vi "LoadFromINI.vi"(8 "error in (no error)":errorcluster, 10 "path":path, 11 "reference in":refnum<class "niMmWave_Reciever.lvclass">) -> (0 "error out":errorcluster, 3 "reference out":refnum<class "niMmWave_Reciever.lvclass">)   [LabVIEW 2019, in "niMmWave_Reciever.lvclass"]
doc: "Loads insturment data from ini file"
uses:
  niMmWave_Reciever.lvclass
  <vilib>/Utility/error.llb/Error Cluster From Error Code.vi
  <vilib>/Utility/config.llb/Read Key (String).vi
  <vilib>/ErrorRing/Error Ring.xnode
  <vilib>/Utility/config.llb/NI_LVConfig.lvlib
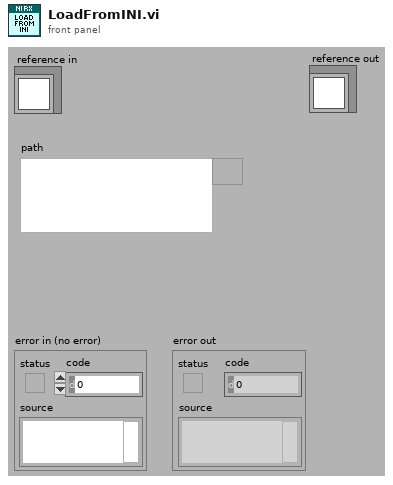
[diagram p1: front panel]
types:
  T1 = cluster{"IF":string, "RX_ADC":string, "RX_FPGA":string}
  T2 = typedef "niMmWave_Reciever.lvclass/ObjectAttributesRef.ctl" = refnum<data-value>
  T3 = typedef "NI_LVConfig.lvlib/Config Data RefNum.ctl" = refnum<k1>
  T4 = typedef "niMmWave_Reciever.lvclass/ObjectAttributes.ctl" = cluster{"session":T5[], "HW.RX devices":T19, "RF config":T20, "RX trigger options":T21, "RX samples":i32, "RX Fs":dbl}
  T5 = typedef "Session.ctl" = cluster{"3620 session":refnum<queue>, "tx baseband session":T6, "rx baseband session":T14, "tx gain (dB)":dbl, "rx gain (dB)":dbl, "hardware configuration":T15, "gain ranging":T17[], "pxi trigger bus information":T18}
  T6 = typedef "Tx Baseband Session.ctl" = cluster{"3610 session":T7, "7902 reference":T13}
  T7 = typedef "ni3610_and_ni3630_Driver_Lib.lvlib/Main Settings.ctl" = cluster{"VISA resource name":refnum<visa-resource-name>, "Address Space":T8, "window_offset":u32, "register_addresses":T9, "required_MM_fpga_version":cluster{"signature":u32, "hardware":u32, "current revision":u32, "oldest revision":u32}, "CPLD Oldest Compat Version ":cluster{"hardware":u32, "CPLD firmware":u32}, "MM_FPGA_image_location":string, "is_init":bool, "card_type":T10, "DacLmkConfigFileName":string, "AdcLmkConfigFileName":string, "AdcConfigFileName":string, "DacConfigFileName_RevA":string, "DacConfigFileName_RevB":string, "Mulde hardware revision":u8, "bypass DAC PLL\n":bool, "IQ Card Revision":T11, "board capability":T12}
  T8 = typedef "VISA Register Access Address Space.ctl" = u16
  T9 = typedef "ni3610_and_ni3630_Driver_Lib.lvlib/Register Adresses.ctl" = cluster{"MM based Registers":cluster{"Revision":u32, "OldestCompatRev":u32, "signature":u32, "scratch":u32, "LedControl":u32, "BoardHwRev":u32, "BoardControl":u32, "ThermalStatus":u32, "BasebandStatus":u32, "BasebandControl":u32, "BasebandAuxSetup":u32, "BasebandAuxStatus":u32, "LmkSyncOutSetup":u32, " AdcSyncOutSetup":u32, " InjSyncOutSetup":u32, " PxiTrig0OutSetup":u32, " PxiTrig1OutSetup":u32, " PxiTrig2OutSetup":u32, " PxiTrig3OutSetup":u32, " PxiTrig4OutSetup":u32, " PxiTrig5OutSetup":u32, " PxiTrig6OutSetup":u32, " PxiTrig7OutSetup":u32}, "CPLD based Registers":cluster{"SlaveSignature":u32, "SlaveRevision":u32, "SlaveOldestCompatRev":u32, "SlaveScratch":u32, "SlaveSetup":u32, "SlaveStatus":u32, "IDacReg_offset":u32, "LMKRegGrp0_offset":u32, "QDacReg_offset":u32, "BrdTempSensorVal":u32, "TempSensorPowerDown":u32, "GPIOReg_offset":u32, "IAdcReg_offset":u32, "QAdcReg_offset":u32, "LMKRegGrp1_offset":u32, "QadcTempSensorVal":u32, "IadcTempSensorVal":u32, "RevisionReg":u32, "VcxoReg":u32, "CpldStatusReg":u32, "PowerReg":u32, "VBiasEnReg":u32, "ExtRefOeReg":u32, "QdacCtrlReg":u32, "QdacStatusReg":u32, "IdacCtrlReg":u32, "IdacStatusReg":u32, "QdacJtagIn":u32, "QdacJtagOut":u32, "IdacJtagIn":u32, "IdacJtagOut":u32, "IqDcSetupReg":u32, "QadcStatusReg":u32, "IadcStatusReg":u32, "BrdSetupReg":u32, "IqDcRevisionReg":u32, "PllStatusReg":u32, "EndpointScratchReg":u32, "AdcSyncCfgReg":u32, "IqCardOpampReg":u32}, "CPLD Register Offset":u32, "MM  Register Offset":u32, " PxiTrig0OutSetup":u32}
  T10 = typedef "ni3610_and_ni3630_Driver_Lib.lvlib/Base Card Type.ctl" = enum16{"unspecified", "ADC", "DAC"}
  T11 = typedef "ni3610_and_ni3630_Driver_Lib.lvlib/IQ Card Revision.ctl" = enum16{"RevA", "RevB", "RevC", "RevD"}
  T12 = typedef "ni3610_and_ni3630_Driver_Lib.lvlib/Board Capability.ctl" = cluster{"baseband sync":enum16{"no baseband sync", "baseband sync"}}
  T13 = typedef "Blank FPGA Reference.ctl" = refnum<k20>
  T14 = typedef "Rx Baseband Session.ctl" = cluster{"3630 session":T7, "7902 reference":T13}
  T15 = typedef "Hardware Configuration.ctl" = cluster{"direction":T16, "baseband only":bool}
  T16 = typedef "Direction.ctl" = enum16{"Transceiver", "Receiver", "Transmitter"}
  T17 = typedef "Gain Ranging.ctl" = cluster{"gain ranging active scope":string, "gain ranging stream session":refnum<k20>}
  T18 = typedef "PXI Trigger Bus Info.ctl" = cluster{"chassis resource name":refnum<visa-resource-name>, "7902R (TX)":i16, "3610 (TX)":i16, "3620 (IF)":i16, "3630 (RX)":i16, "7902R (RX)":i16}
  T19 = typedef "mmWave HW Control.lvlib/HW RX resources cluster.ctl" = cluster{"HW.IF":tag, "HW.ADC":refnum<visa-resource-name>, "HW.RX FPGA":tag}
  T20 = typedef "mmWave HW Control.lvlib/HW RX RF config cluster.ctl" = cluster{"Gain":dbl, "Frequency":dbl, "mmWave adapter":string}
  T21 = typedef "TX trigger config.ctl" = cluster{"delay":dbl, "trig source":T22, "PXI src":i32, "export":T23, "PXI dest":i32}
  T22 = typedef "FPGA Utility.lvlib/FPGA driver trigger source.ctl" = enum16{"Use Tclk", "PXI_Trig", "Aurora RX trig"}
  T23 = typedef "FPGA Utility.lvlib/FPGA driver trigger destination.ctl" = enum16{"None", "Source trig", "Synced trig", "Delayed sync"}
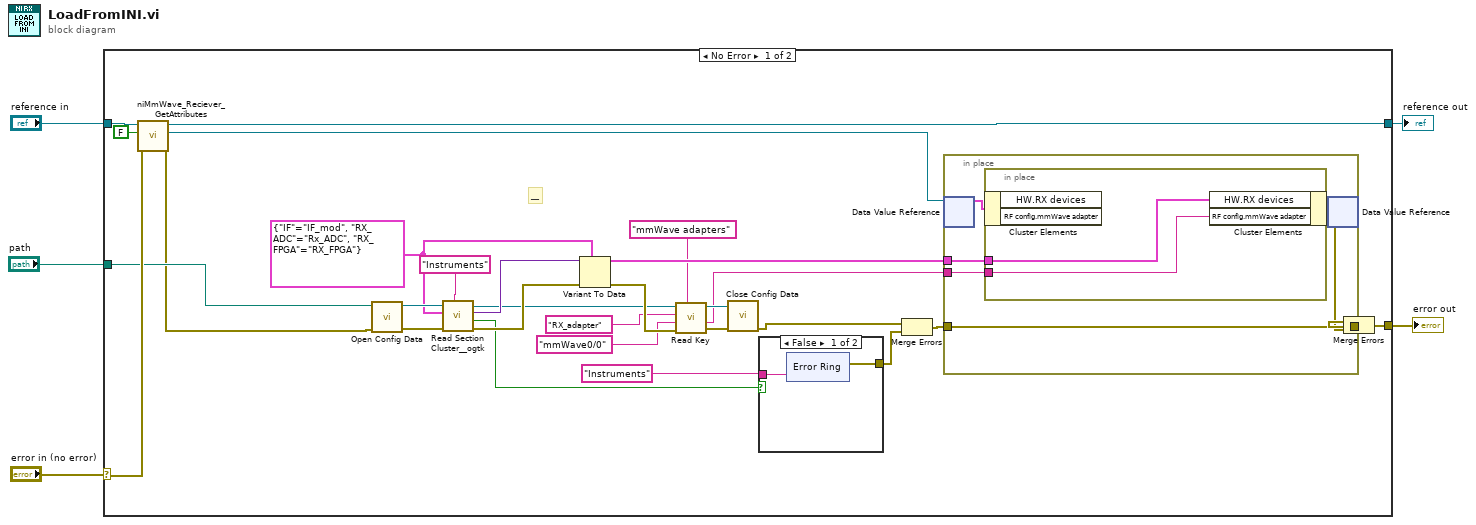
[diagram p0: block diagram]
diagram:
  n1 = case shown="No Error" "error in (no error)" {
    selector: "error in (no error)" -> [w32 w53]
    tunnel: [w35 w53] -> w4
    tunnel: [w33 w52] -> w2
    tunnel: "reference in" -> [w34 w52]
    tunnel: "path" -> [w21 _]
    frame No Error {
      w22 = T1 {"IF"="IF_mod", "RX_ADC"="Rx_ADC", "RX_FPGA"="RX_FPGA"} ("HW.RX resources")
      # "__"
      n2 = call "niMmWave_Reciever_GetAttributes.vi"("error in (no error)"=w32, "return data? (T)"=FALSE, "reference in"=w34) -> ("error out"=w14:errorcluster, "attributes ref"=w29:T2, "reference out"=w33:refnum<class "niMmWave_Reciever.lvclass">)  [unwired: 5 in, 1 out]
      n3 = call <vilib>:"Open Config Data.vi"("error in (no error)"=w14, "configuration file path"=w21) -> ("error out"=w26:errorcluster, "refnum"=w27:T3)  [unwired: 7 in, 1 out]
      n4 = call <userlib>:"Read Section Cluster__ogtk.vi"("section (optional)"="Instruments", "error in (no error)"=w26, "Section Formatted Cluster Type"=w22, "refnum"=w27) -> ("error out"=w24:errorcluster, "all found?"=w20:bool, "Section Formatted Cluster"=w25:variant, "dup refnum"=w11:T3)  [unwired: 3 in, 1 out]
      n5 = Variant To Data(error in=w24, type=w22, Variant=w25) -> (data=w17:T1, error out=w13:errorcluster)
      n6 = call-poly <vilib>:"Read Key.vi"("section"="mmWave adapters" ("section (optional)"), "error in (no error)"=w13, "default value"="mmWave0/0" ("section (optional)"), "key"="RX_adapter" ("section (optional)"), "refnum"=w11) -> ("error out"=w8:errorcluster, "value"=w7:string, "refnum out"=w9:T3)  [unwired: 3 in, 1 out]
      n7 = call <vilib>:"Close Config Data.vi"("error in (no error)"=w8, "refnum"=w9) -> ("error out"=w16:errorcluster)  [unwired: 8 in, 1 out]
      n8 = case shown="False" w20 {
        tunnel: "Instruments" ("section (optional)") -> [w44 _]
        tunnel: [w43 _] -> w18
        frame False {
          n9 = xnode "Error Ring"("parameter 0"=w44) -> ("error out"=w43:errorcluster)
        }
        frame True {
        }
      }
      n10 = Merge Errors(w16, w18) -> (w15:errorcluster)
      n11 = in-place {
        in-place-border: w15 -> [w38]
        in-place-border: [w38] -> w31
        in-place-border: w17 -> [w37]
        in-place-border: w7 -> [w36]
        n12 = in-place-dvr #1(w29) -> (w39:T4)  [unwired: 1 out]
        n13 = in-place {
          in-place-border: w37 -> [w42]
          in-place-border: w36 -> [w41]
          n14 = in-place-cluster #2(w39) -> ()  [unwired: 2 out]
          n15 = in-place-cluster #2("HW.RX devices"=w42, "RF config.mmWave adapter"=w41) -> (w40:T4)
        }
        n16 = in-place-dvr #1(w40) -> (w30:errorcluster)  [unwired: 1 out]
      }
      n17 = Merge Errors(w31, w30) -> (w35:errorcluster)
    }
    frame Error {
    }
  }
  "error out" <- w4
  "reference out" <- w2
